vi "LogFFT without Windowing.vi"(5 "FFT Pad?":bool, 9 "Padded FT Size":i32, 10 "FFT {X}":cdb[](array[numeric])) -> (2 "Log{Mag(FFT)}":dbl[](array[numeric]))   [LabVIEW 2012]
uses:
  <vilib>/Analysis/2dsp.llb/Inverse Complex FFT.vi
  <vilib>/Analysis/NI_AALPro.lvlib
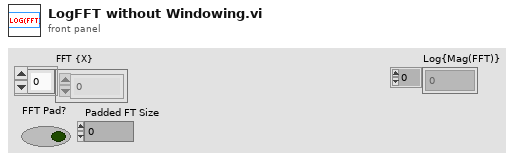
[diagram p1: front panel]
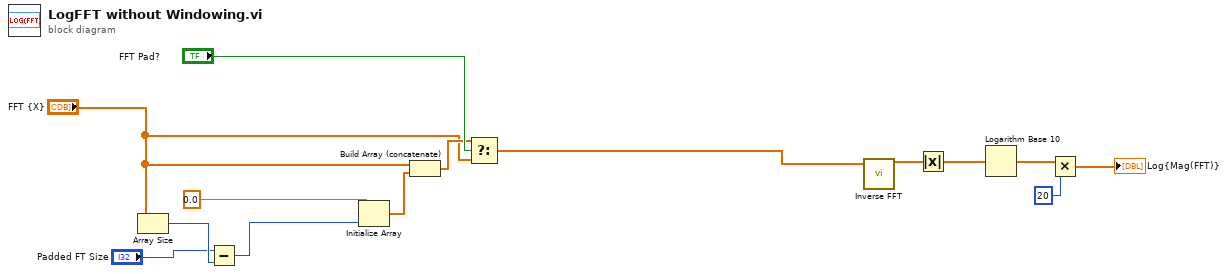
[diagram p0: block diagram]
diagram:
  n1 = Array Size(array="FFT {X}") -> (size(s)=w6:i32)
  n2 = Subtract(x="Padded FT Size", y=w6) -> (x-y=w4:i32)
  n3 = Initialize Array(0.0 ("element"), w4) -> (w9:dbl[])
  n4 = Build Array (concatenate)("FFT {X}", w9) -> (w7:cdb[])
  n5 = Select(t=w7, s="FFT Pad?", f="FFT {X}") -> (s? t:f=w1:cdb[])
  n6 = call-poly <vilib>:"Inverse FFT.vi"("FFT {X}"=w1) -> ("X"=w3:cdb[])  [unwired: 9 in, 1 out]
  n7 = Absolute Value(x=w3) -> (abs(x)=w11:dbl[])
  n8 = Logarithm Base 10(1:w11) -> (0:w14:dbl[])
  n9 = Multiply(x=w14, y=20) -> (x*y=→"Log{Mag(FFT)}":dbl[])
